vi "fn Connect.vi"(8 "error in (no error)":errorcluster, 11 "server_id":i32) -> (0 "error out":errorcluster, 3 "function return":i32)   [LabVIEW 2024, in "LV_OPC.lvlib"]
doc: "LVOPC_API int fnConnect(int server_id);"
uses:
  LV_OPC.lvlib
  LVOPC64.dll
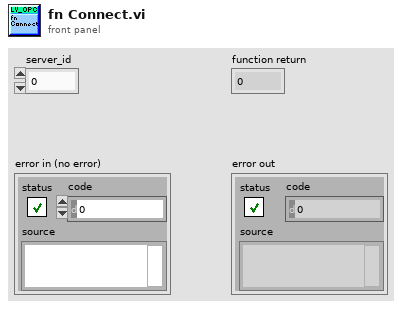
[diagram p1: front panel]
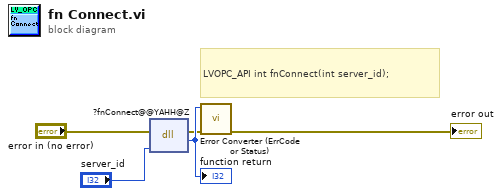
[diagram p0: block diagram]
diagram:
  # "LVOPC_API int fnConnect(int server_id);"
  n1 = dll-call lib="C:/Users/Andrey/Desktop/LV_OPC-Client-x64/LV_OPC_Test/OPC.DLL/LVOPC64.*" fn="?fnConnect@@YAHH@Z"(error in="error in (no error)", "server_id"="server_id") -> (error out=w2:errorcluster, "return type"=w5:i32)  [unwired: 3 in, 1 out]
  "function return" <- w5
  n2 = call "Error Converter (ErrCode or Status).vi"("error in (no error)"=w2, "error code"=w5) -> ("error out"=→"error out":errorcluster)  [unwired: 9 in]
